vi "Check in Map.vi"(8 "error in (no error)":errorcluster, 9 "lower limit":dbl, 10 "upper limit":dbl, 11 "Cave in":refnum<class "Cave.lvclass">) -> (0 "error out":errorcluster, 2 "in Map?":bool, 3 "Cave out":refnum<class "Cave.lvclass">)   [LabVIEW 2023, in "d15.lvlib" / "Cave.lvclass"]
uses:
  Cave.lvclass
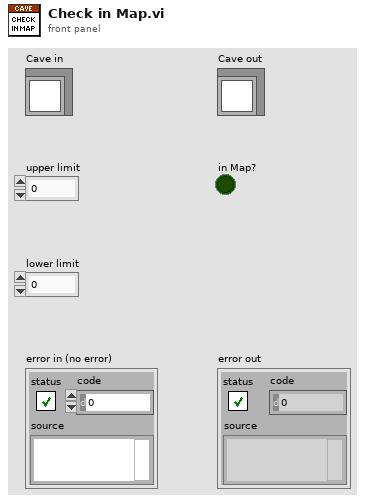
[diagram p1: front panel]
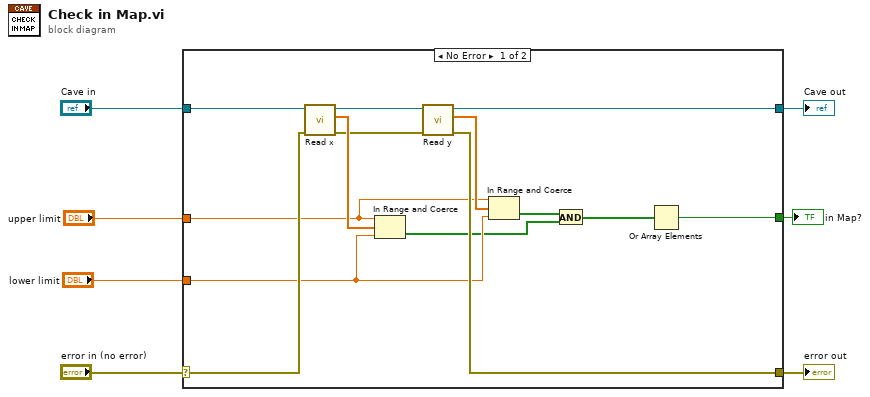
[diagram p0: block diagram]
diagram:
  n1 = case shown="No Error" "error in (no error)" {
    selector: "error in (no error)" -> [w19 w23]
    tunnel: [w15 w23] -> w6
    tunnel: [w17 w22] -> w4
    tunnel: "Cave in" -> [w20 w22]
    tunnel: "upper limit" -> [w13 _]
    tunnel: "lower limit" -> [w12 _]
    tunnel: [w8 _] -> w1
    frame No Error {
      n2 = call-dynamic "Read x.vi"("error in (no error)"=w19, "Diamond in"=w20) -> ("error out"=w16:errorcluster, "x"=w21:dbl[], "Diamond out"=w18:refnum<class "Cave.lvclass">)  [unwired: 7 in]
      n3 = In Range and Coerce(upper limit=w13, x=w21, lower limit=w12) -> (In Range?=w10:bool[])  [unwired: 1 out]
      n4 = call-dynamic "Read y.vi"("error in (no error)"=w16, "Diamond in"=w18) -> ("error out"=w15:errorcluster, "y"=w14:dbl[], "Diamond out"=w17:refnum<class "Cave.lvclass">)  [unwired: 7 in]
      n5 = In Range and Coerce(upper limit=w13, x=w14, lower limit=w12) -> (In Range?=w11:bool[])  [unwired: 1 out]
      n6 = And(x=w11, y=w10) -> (x .and. y?=w9:bool[])
      n7 = Or Array Elements(Boolean array=w9) -> (logical OR=w8:bool)
    }
    frame Error {
    }
  }
  "error out" <- w6
  "Cave out" <- w4
  "in Map?" <- w1
